vi "Actor Core.vi"(8 "error in":errorcluster, 11 "Logger in":refnum<class "Logger.lvclass">) -> (0 "error out":errorcluster, 3 "Actor out":refnum<class "Actor.lvclass">)   [LabVIEW 2020, in "CANopen Logging.lvlib" / "Logger.lvclass"]
doc: "<p>(<strong>Filename</strong>: <span class=\"dnl\">Actor Framework.lvlib:Actor.lvclass:Actor Core.vi</span>)</p>\n<p>Receives messages to the actor, reacts to them, and initiates any error handling that may shut the actor down.</p>\n<p>Descendant classes may override this VI to append parallel tasks for the actor to complete while it handles messages. Overrides use the <a href=\"nihelplauncher://docs/csh?context=lvcore_glang_udclass\">Call Parent Class Method</a> node.</p>"
uses:
  Logger.lvclass
  <vilib>/ActorFramework/Actor/Actor.lvclass
  Logger.lvclass/Logger.ctl
  HAL/Source/Interfaces/IMessage/IMessage.lvclass
  Log Level.vi
  CANopen Logging.lvlib
  <vilib>/Utility/SystemLogging/NI_SystemLogging.lvlib
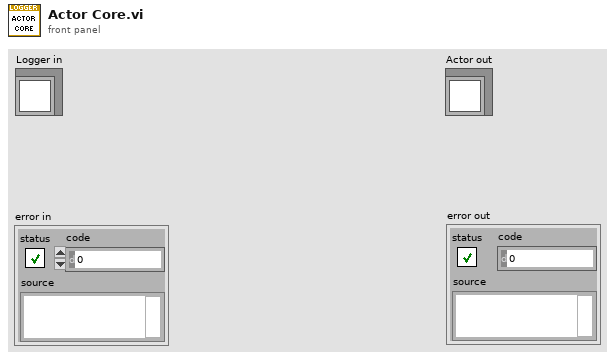
[diagram p1: front panel]
types:
  T1 = enum16{"Error", "Warn", "Info", "Debug", "Trace"}
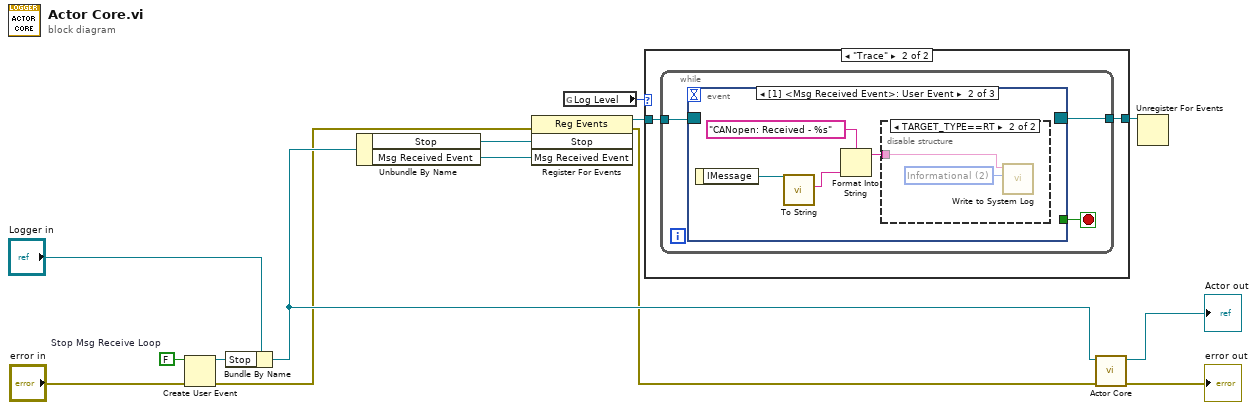
[diagram p0: block diagram]
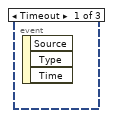
[diagram p3: hidden frame]
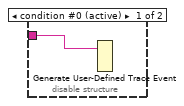
[diagram p4: hidden frame]
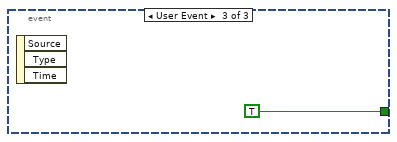
[diagram p5: hidden frame]
diagram:
  w12 = FALSE  # Stop Msg Receive Loop
  n1 = Create User Event(user event datatype=w12, error in="error in") -> (user event=w7:refnum<user-event>, error out=w5:errorcluster)
  n2 = Bundle By Name(cluster="Logger in", "Stop"=w7) -> (w6:refnum<class "Logger.lvclass">)
  n3 = Unbundle By Name(w6) -> ("Stop"=w11:refnum<user-event>, "Msg Received Event"=w9:refnum<user-event>)
  n4 = register-events(error in=w5, w11, w9) -> (reference out=w3:refnum<event-registration>, error out=w1:errorcluster)  [unwired: 1 in]
  n5 = global read "Log Level.vi" "Log Level"() -> (w2:T1)
  n6 = case shown="\"Trace\"" w2 {
    tunnel: [w15 w17] -> w4
    tunnel: w3 -> [w15 w16]
    frame Default {
    }
    frame "Trace" {
      n7 = while {
        tunnel: w16 -> [w20]
        tunnel: [w18] -> w17
        stop <- w19 stop-if-true
        n8 = event shown="[1] <Msg Received Event>: User Event" {
          selector: w20 -> [_ _ _]
          dyn-events: [_ _ _] -> w18
          timeout: _ -> [_ _ _]
          tunnel: [_ _ TRUE] -> w19
          event Timeout {
            n9 = event-data() -> ()  [unwired: 1 in, 3 out]
          }
          event User Event {
            n10 = event-data() -> ("IMessage"=w24:refnum<class "IMessage.lvclass">)  [unwired: 1 in]
            n11 = call-dynamic "To String.vi"("IMessage in"=w24) -> ("Stringified"=w22:string)  [unwired: 8 in, 2 out]
            n12 = Format Into String(format string="CANopen: Received - %s", w22) -> (resulting string=w21:string)  [unwired: 2 in, 1 out]
            n13 = disable-structure shown="TARGET_TYPE==RT" {
              disable-tunnel: w21 -> [w25 w27]
              frame condition #0 (active) {
                n14 = Generate User-Defined Trace Event(2:w25) -> ()  [unwired: 1 in]
              }
              frame condition #1 {
                w26 = 2 items=["Error", "Warning", "Informational"] ("severity")
                n15 = call <vilib>:"Write to System Log.vi"("severity"=w26, "message"=w27) -> ()  [unwired: 9 in, 1 out]
              }
            }
          }
          event User Event {
            n16 = event-data() -> ()  [unwired: 1 in, 3 out]
          }
        }
      }
    }
  }
  n17 = call-parent "Actor Core.vi"("error in"=w1, "Actor in"=w6) -> ("error out"=→"error out":errorcluster, "Actor out"=→"Actor out":refnum<class "Actor.lvclass">)  [unwired: 8 in]
  n18 = Unregister For Events(event registration refnum=w4) -> ()  [unwired: 1 in, 1 out]
